vi "SeCrTs-TC_Read.vi"(8 "error in (no error)":errorcluster, 9 "Numeric":dbl, 10 "TC_Task":refnum<k21>, 11 "Data FIFO Ref":T1) -> (0 "error out":errorcluster, 2 "task out":refnum<k21>)   [LabVIEW 2022 SP3]
uses:
  RT Controls/SeCrTs-Data FIFO.ctl
  <vilib>/Platform/TimedLoop/XDataNode/timing_clust.ctl
  <vilib>/Platform/TimedLoop/XDataNode/nitl_modes.ctl
  <vilib>/Platform/TimedLoop/XDataNode/wakeup.ctl
  <vilib>/Analysis/3filter.llb/Filter Structure Type.ctl
  <vilib>/DAQmx/read.llb/DAQmx Read (Analog 1D Wfm NChan NSamp).vi
  <vilib>/DAQmx/miscellaneous.llb/DAQmx Fill In Error Info.vi
  <vilib>/measure/macond.llb/IIR Filter for N Chan.vi
  <vilib>/platform/TimedLoop/XDataNode/XDataNode.xnode
  <vilib>/Platform/TimedLoop/XDataNode/XDNodeRunTimeDep.lvlib
  <vilib>/measure/NI_MAPro.lvlib
  <vilib>/Analysis/NI_AALBase.lvlib
  RT Controls/ATF Storage Haelth.ctl
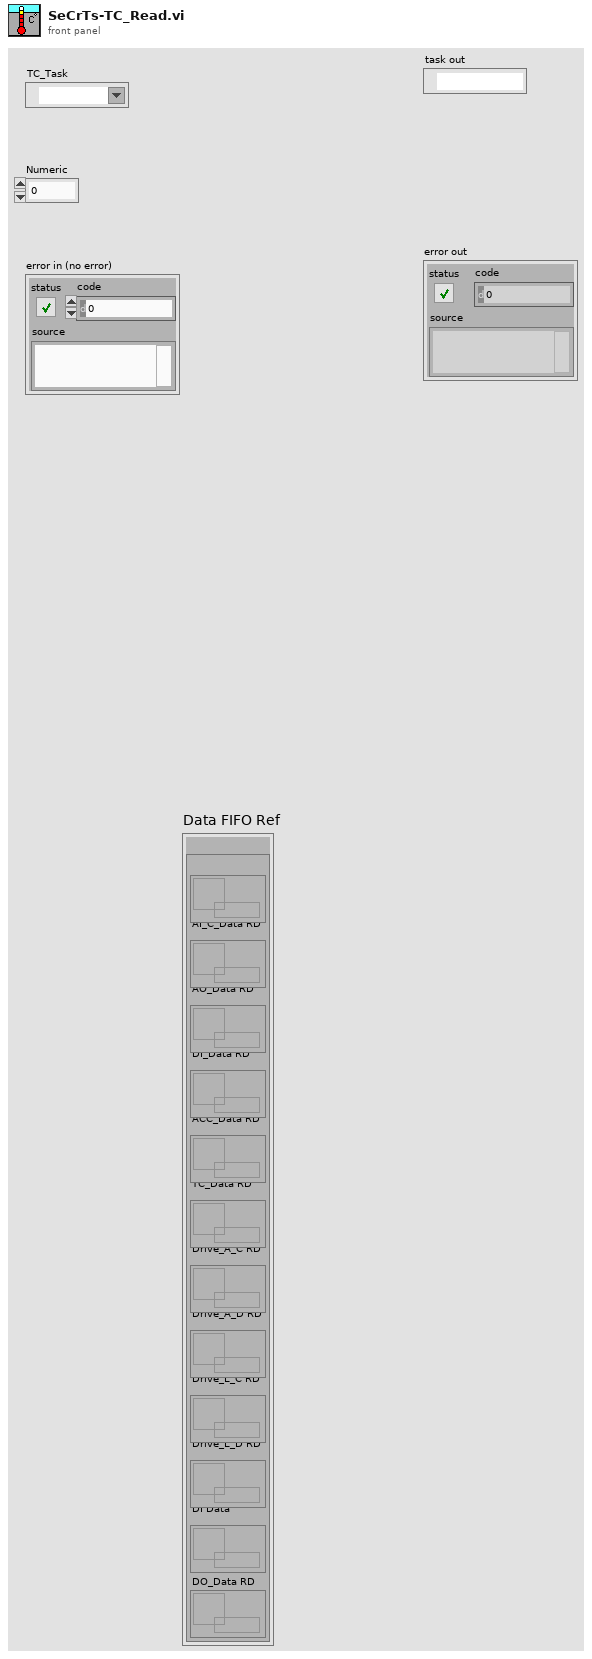
[diagram p1: front panel]
types:
  T1 = typedef "SeCrTs-Data FIFO.ctl" = cluster{"RD":cluster{"AI_V_Data RD":refnum<queue>, "AI_C_Data RD":refnum<queue>, "AO_Data RD":refnum<queue>, "DI_Data RD":refnum<queue>, "ACC_Data RD":refnum<queue>, "TC_Data RD":refnum<queue>, "Drive_A_C RD":refnum<queue>, "Drive_A_D RD":refnum<queue>, "Drive_L_C RD":refnum<queue>, "Drive_L_D RD":refnum<queue>, "DI Data":refnum<queue>, "DO_Data RD":refnum<queue>}}
  T2 = typedef "XDNodeRunTimeDep.lvlib/timing_clust.ctl" = cluster{"Expected End [f-1]":u64, "Actual End [f-1]":u64, "Finished Late? [f-1]":bool, "Expected End [i-1]":u64, "Actual End [i-1]":u64, "Finished Late? [i-1]":bool, "Expected Start [i]":u64, "Actual Start [i]":u64, "Expected Start [f]":u64, "Actual Start [f]":u64, "Source Name":string, "Structure Name":string, "Period":i64, "Deadline":i64, "Offset":i64, "Start":i64, "Priority":i32, "Timeout":i32, "Mode":T3, "Wakeup Reason":T4, "Error":errorcluster, "Source Type":string, "Secondary Source Type":string, "Global End Time":u64, "Global Start Time":u64, "Frame Duration":u64, "Iteration Duration":u64, "Assigned CPU":i32, "I/O Scan Engine Mode":u32}
  T3 = typedef "XDNodeRunTimeDep.lvlib/nitl_modes.ctl" = enum32{"No Change", "Process missed periods, maintain original phase", "Discard missed periods, maintain original phase", "Process missed periods, ignore original phase", "Discard missed periods, ignore original phase"}
  T4 = typedef "XDNodeRunTimeDep.lvlib/wakeup.ctl" = enum32{"Normal", "Aborted", "Asynchronous wakeup", "Timing source error", "Timed loop error", "Timeout"}
  T5 = typedef "ATF Storage Haelth.ctl" = enum16{"AI C", "AI V", "AO", "DI", "DO", "TC", "ACC", "RT Str", "DR A"}
  T6 = cluster{"Topology":enum16{"Off", "Butterworth", "Chebyshev", "Inverse Chebyshev", "Elliptic", "Bessel"}, "Type":enum16{"Lowpass", "Highpass", "Bandpass", "Bandstop"}, "Order":i32, "Lower Fc":dbl, "Upper Fc":dbl, "PB Ripple":dbl, "SB Attenuation":dbl}
  T7 = enum16{"Init", "Read 'All'", "Read 'n'", "Read '1'", "Write '1'", "Write 'n'", "Write 'All'"}
  T8 = typedef "NI_AALBase.lvlib/Filter Structure Type.ctl" = u16
  T9 = cluster{"Start DAQ":bool, "Stop DAQ":bool, "RT Stop":bool, "RT Exit":bool, "Start Seq":bool}
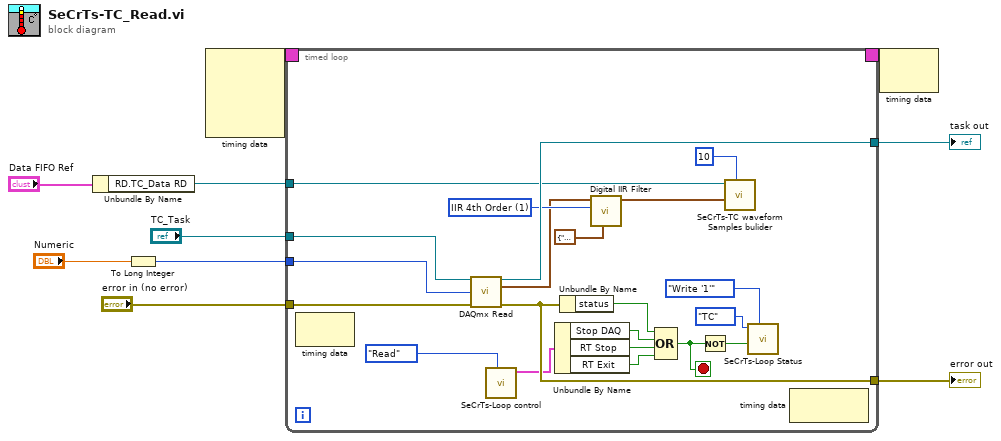
[diagram p0: block diagram]
diagram:
  n1 = Unbundle By Name("Data FIFO Ref") -> ("RD.TC_Data RD"=w1:refnum<queue>)
  n2 = To Long Integer(number="Numeric") -> (32bit integer=w5:i32)
  n3 = node-c288() -> (w4:T2)  [unwired: 4 in]
  n4 = timed-loop {
    tunnel: "error in (no error)" -> [w31]
    tunnel: "TC_Task" -> [w30]
    tunnel: w5 -> [w29]
    tunnel: [w28] -> w6
    tunnel: [w27] -> w10
    timing: w4 -> [_]
    timing-out: [_] -> w3
    tunnel: w1 -> [w17]
    stop <- w19 stop-if-true
    w15 = T8 1 items=["IIR 2nd Order"=0, "IIR 4th Order"=1, "Auto Select"=10] ("filter structure option")
    n5 = node-c288() -> ()  [unwired: 1 in, 1 out]
    n6 = call-poly <vilib>:"DAQmx Read.vi"("task/channels in"=w30, "number of samples per channel"=w29, "error in"=w31) -> ("task out"=w27:refnum<k21>, "data"=w13:waveform(dbl)[], "error out"=w28:errorcluster)  [unwired: 10 in]
    n7 = call "SeCrTs-Loop control.vi"("Action"=enum16{"Init", "Write", "Read"}."Read") -> ("Loop Control out"=w25:T9)  [unwired: 9 in, 1 out]
    n8 = Unbundle By Name(w25) -> ("Stop DAQ"=w24:bool, "RT Stop"=w23:bool, "RT Exit"=w22:bool)
    n9 = Unbundle By Name(w28) -> ("status"=w26:bool)
    n10 = call-poly <vilib>:"Digital IIR Filter.vi"("IIR filter specifications"=T6 {"Topology"=enum."Butterworth", "Type"=enum."Lowpass", "Order"=4, "Lower Fc"=1.0, "Upper Fc"=200.0, "PB Ripple"=1.0, "SB Attenuation"=60.0}, "filter structure option"=w15, "signal(s) in"=w13) -> ("signal(s) out"=w12:waveform(dbl)[])  [unwired: 6 in, 2 out]
    n11 = Compound Arithmetic op=OR(w26, w24, w23, w22) -> (w19:bool)
    n12 = Not(x=w19) -> (.not. x?=w20:bool)
    n13 = call "SeCrTs-TC waveform Samples bulider .vi"("Samples"=10, "Data input"=w12, "RD.TC_Data RD"=w17) -> ()  [unwired: 8 in, 1 out]
    n14 = call "SeCrTs-Loop Status.vi"("Option"=T7."Write '1'", "Status"=w20, "Loop"=ATF_Storage_Haelth."TC") -> ()  [unwired: 6 in, 3 out]
    n15 = node-c288() -> ()  [unwired: 1 in, 1 out]
  }
  "task out" <- w10
  "error out" <- w6
  n16 = node-c288(w3) -> ()  [unwired: 1 out]
